vi "索引数据并插入.vi"(8 "error in (no error)":errorcluster, 9 "数据类别":enum16{"水样数据", "日质控数据"}(ring), 10 "索引记录":timestamp format="%<%H:%M:%S\n%m/%d/%Y>T", 11 "table":string) -> (0 "error out":errorcluster, 3 "最新索引记录":timestamp)   [LabVIEW 2016, in "数据查询.lvlib"]
uses:
  <vilib>/addons/database/Connection.llb/DB Tools Open Connec (String).vi
  <vilib>/addons/database/_DB Variant To Data/Database Variant To Data.xnode
  <vilib>/addons/database/NI_Database_API.lvlib
panel:
  in  "data in":cluster{"时间":timestamp, "测量模式":string, "值":sgl}
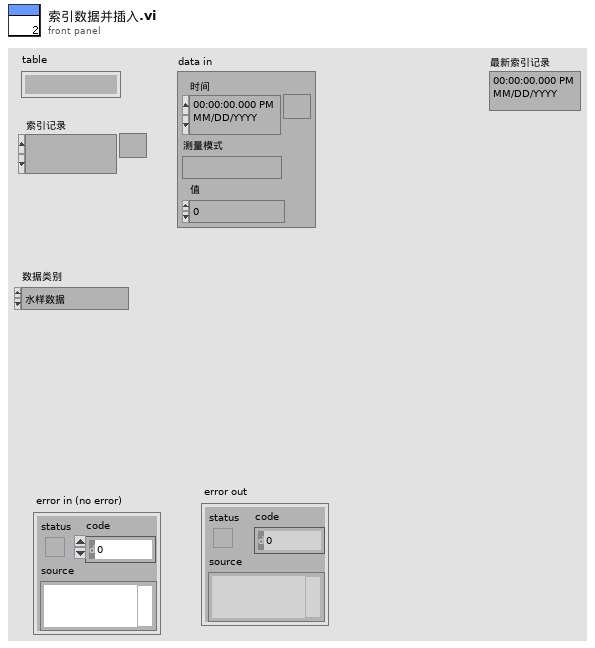
[diagram p1: front panel]
types:
  T1 = typedef "数据库类型.ctl" = enum16{"Access", "SQLite"}
  T2 = cluster{"时间":timestamp, "测量模式":string, "值":sgl}[]
  T3 = typedef "NI_Database_API.lvlib/Conn ObjectReference.ctl" = refnum<k1>
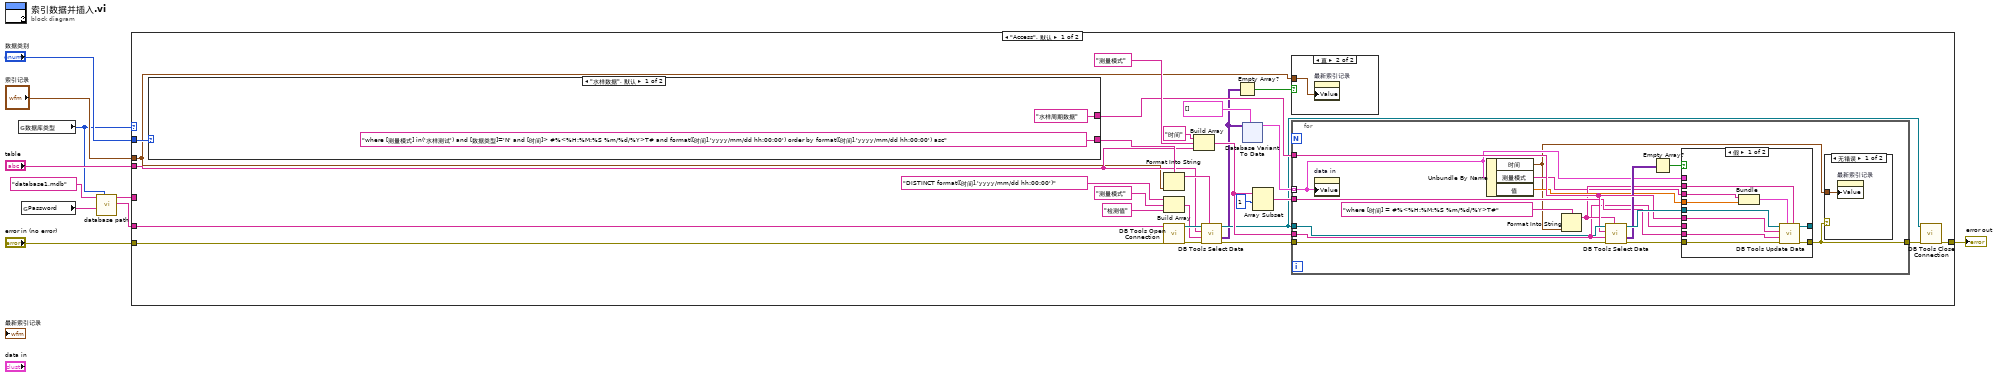
[diagram p0: block diagram]
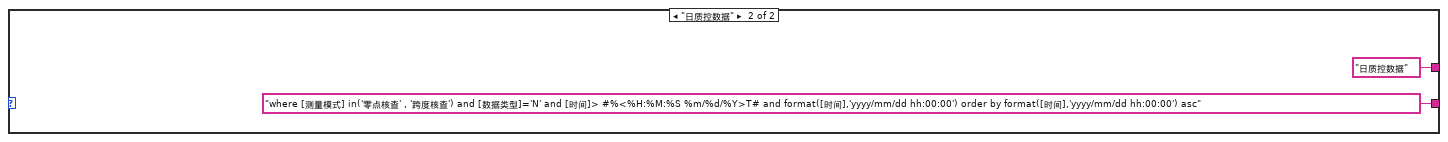
[diagram p3: hidden frame]
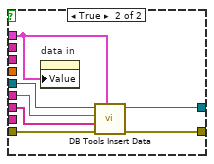
[diagram p5: hidden frame]
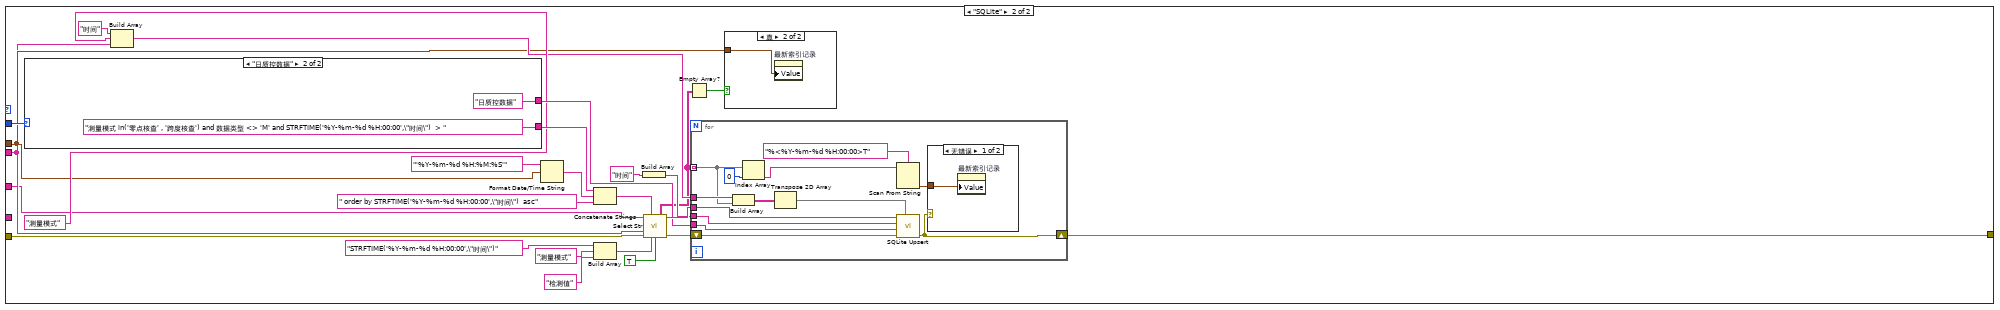
[diagram p6: hidden frame]
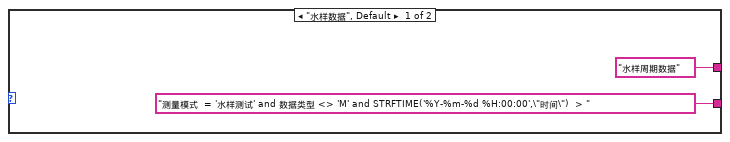
[diagram p9: hidden frame]
diagram:
  n1 = global read "全局变量.vi" "数据库类型"() -> (w4:T1)
  n2 = global read "全局变量.vi" "Password"() -> (w1:string)
  n3 = call "database path.vi"("数据库类型"=w4, "Password"=w1, "database"="database1.mdb") -> ("Connection information"=w2:string, "Path out"=w3:string)  [unwired: 7 in]
  n4 = case shown="\"Access\", 默认" w4 {
    tunnel: "索引记录" -> [w13 w195]
    tunnel: "error in (no error)" -> [w28 w217]
    tunnel: [w27 w201] -> w6
    tunnel: "数据类别" -> [w21 w218]
    tunnel: "table" -> [w20 w194]
    tunnel: w3 -> [_ w193]
    tunnel: w2 -> [w11 _]
    frame "Access", Default {
      n5 = case shown="\"水样数据\", 默认" w21 {
        tunnel: ["where [测量模式] in('水样测试') and [数据类型]='N' and [时间]> #%<%H:%M:%S %m/%d/%Y>T# and format([时间],'yyyy/mm/dd hh:00:00') order by format([时间],'yyyy/mm/dd hh:00:00') asc" ("condition") "where [测量模式] in('零点核查' , '跨度核查') and [数据类型]='N' and [时间]> #%<%H:%M:%S %m/%d/%Y>T# and format([时间],'yyyy/mm/dd hh:00:00') order by format([时间],'yyyy/mm/dd hh:00:00') asc" ("condition")] -> w23
        tunnel: ["水样周期数据" "日质控数据"] -> w22
        frame "水样数据", Default {
        }
        frame "日质控数据" {
        }
      }
      n6 = Format Into String(format string=w23, w13) -> (resulting string=w33:string)  [unwired: 2 in, 1 out]
      n7 = Build Array("DISTINCT format([时间],'yyyy/mm/dd hh:00:00')", "测量模式" ("元素"), "检测值" ("元素")) -> (w32:string[])
      n8 = call-poly <vilib>:"DB Tools Open Connection.vi"("error in (no error)"=w28, "connection information"=w11) -> ("error out"=w34:errorcluster, "connection reference"=w35:T3)  [unwired: 6 in]
      n9 = Build Array("时间", "测量模式" ("元素"), w20) -> (w31:string[])
      n10 = call <vilib>:"DB Tools Select Data.vi"("condition"=w33, "error in (no error)"=w34, "columns"=w32, "table"=w20, "connection reference"=w35) -> ("error out"=w16:errorcluster, "data"=w14:variant[][], "connection reference out"=w17:T3)  [unwired: 1 in]
      n11 = Empty Array?(array=w14) -> (empty?=w12:bool)
      n12 = xnode "Database Variant To Data"("database variant"=w14, "type"=T2 []) -> ("data"=w18:T2)  [unwired: 1 in, 1 out]
      n13 = Array Subset(array=w31, index=1 ("索引")) -> (w29:string[])  [unwired: 1 in]
      n14 = case shown="真" w12 {
        tunnel: w13 -> [_ w38]
        frame False {
        }
        frame True {
          n15 = property on="最新索引记录" class="AbsTime (严格)"("Value"=w38) -> ()  [unwired: 2 in, 2 out]
        }
      }
      n16 = for {
        tunnel: w18 -> [w45] mode=indexing
        tunnel: w17 -> [w56]
        tunnel: w16 -> [w55]
        tunnel: [w44] -> w15
        tunnel: w22 -> [w52]
        tunnel: w31 -> [w47]
        tunnel: w29 -> [w49]
        n17 = property on="data in" class="Clust (严格)"("Value"=w45) -> ()  [unwired: 2 in, 2 out]
        n18 = Unbundle By Name(w45) -> ("时间"=w43:timestamp, "测量模式"=w46:string, "值"=w50:sgl)
        n19 = Format Into String(format string="where [时间] = #%<%H:%M:%S %m/%d/%Y>T#" ("condition"), w43) -> (resulting string=w48:string)  [unwired: 2 in, 1 out]
        n20 = call <vilib>:"DB Tools Select Data.vi"("condition"=w48, "error in (no error)"=w55, "columns"=w47, "table"=w52, "connection reference"=w56) -> ("error out"=w53:errorcluster, "data"=w51:variant[][], "connection reference out"=w54:T3)  [unwired: 1 in]
        n21 = Empty Array?(array=w51) -> (empty?=w57:bool)
        n22 = case shown="假" w57 {
          tunnel: w52 -> [w65 w76]
          tunnel: w54 -> [w69 w75]
          tunnel: w53 -> [w68 w74]
          tunnel: [w66 w72] -> w44
          tunnel: [w67 w73] -> _
          tunnel: w50 -> [w64 _]
          tunnel: w49 -> [w62 _]
          tunnel: w48 -> [w61 _]
          tunnel: w47 -> [_ w71]
          tunnel: w46 -> [w60 _]
          tunnel: w45 -> [_ w70]
          frame False {
            n23 = Bundle("测量模式"=w60, "值"=w64) -> (w63:cluster{"测量模式":string, "值":sgl})  [unwired: 1 in]
            n24 = call <vilib>:"DB Tools Update Data.vi"("condition"=w61, "data"=w63, "error in (no error)"=w68, "columns"=w62, "table"=w65, "connection reference"=w69) -> ("error out"=w66:errorcluster, "connection reference out"=w67:T3)  [unwired: 4 in]
          }
          frame True {
            n25 = property on="data in" class="Clust (严格)"("Value"=w70) -> ()  [unwired: 2 in, 2 out]
            n26 = call <vilib>:"DB Tools Insert Data.vi"("data"=w70, "error in (no error)"=w74, "columns"=w71, "table"=w76, "connection reference"=w75) -> ("error out"=w72:errorcluster, "connection reference out"=w73:T3)  [unwired: 5 in]
          }
        }
        n27 = case shown="无错误" w44 {
          tunnel: w43 -> [w59 _]
          frame No Error {
            n28 = property on="最新索引记录" class="AbsTime (严格)"("Value"=w59) -> ()  [unwired: 2 in, 2 out]
          }
          frame Error {
          }
        }
      }
      n29 = call <vilib>:"DB Tools Close Connection.vi"("error in (no error)"=w15, "connection reference"=w17) -> ("error out"=w27:errorcluster)  [unwired: 5 in]
    }
    frame "SQLite" {
      n30 = case shown="\"日质控数据\"" w218 {
        tunnel: ["测量模式  = '水样测试' and 数据类型 <> 'M' and STRFTIME('%Y-%m-%d %H:00:00',\"时间\")  > " ("condition") "测量模式 in('零点核查' , '跨度核查') and 数据类型 <> 'M' and STRFTIME('%Y-%m-%d %H:00:00',\"时间\")  > " ("condition")] -> w210
        tunnel: ["水样周期数据" "日质控数据"] -> w204
        frame "水样数据", Default {
        }
        frame "日质控数据" {
        }
      }
      n31 = Build Array("时间", "测量模式" ("元素"), w194) -> (w200:string[])
      n32 = Format Date/Time String(time format string (%c)="'%Y-%m-%d %H:%M:%S'" ("时间格式字符串(%c)"), seconds (now)=w195) -> (date/time string=w209:string)  [unwired: 1 in]
      n33 = Concatenate Strings(w210, w209, " order by STRFTIME('%Y-%m-%d %H:00:00',\"时间\")  asc" ("字符串")) -> (w207:string)
      n34 = Build Array("STRFTIME('%Y-%m-%d %H:00:00',\"时间\")", "测量模式" ("元素"), "检测值" ("元素")) -> (w213:string[])
      n35 = Build Array("时间") -> (w198:string[])
      n36 = call "Select Str.vi"("DB Path"=w193, "Where Clause"=w207, "Tables Name"=w194, "error in (no error)"=w217, "Columns"=w213, "Distinct"=TRUE) -> ("Results"=w197:string[][], "DB Path Out"=w205:string, "error out"=w206:errorcluster)  [unwired: 6 in, 1 out]
      n37 = Empty Array?(array=w197) -> (empty?=w196:bool)
      n38 = for {
        tunnel: w205 -> [w222]
        tunnel: w204 -> [w220]
        tunnel: w197 -> [w229] mode=indexing
        tunnel: w200 -> [w231]
        shift-right: [w224] -> w201
        shift-left: w206 -> [w232]
        tunnel: w198 -> [w221]
        n39 = Build Array(w231, w229) -> (w230:string[][])
        n40 = Index Array(array=w229, index=0 ("索引")) -> (element=w226:string)
        n41 = Transpose 2D Array(2D array=w230) -> (transposed array=w223:string[][])
        n42 = Scan From String(format string="%<%Y-%m-%d %H:00:00>T" ("格式字符串"), input string=w226) -> (output 1=w225:timestamp)  [unwired: 3 in, 3 out]
        n43 = call "SQLite Upsert.vi"("Column/Value Pairs"=w223, "错误输入（无错误）"=w232, "Table Name"=w220, "Constraint Columns"=w221, "DB Path"=w222) -> ("错误输出"=w224:errorcluster)  [unwired: 2 in, 2 out]
        n44 = case shown="无错误" w224 {
          tunnel: w225 -> [w233 _]
          frame No Error {
            n45 = property on="最新索引记录" class="AbsTime (严格)"("Value"=w233) -> ()  [unwired: 2 in, 2 out]
          }
          frame Error {
          }
        }
      }
      n46 = case shown="真" w196 {
        tunnel: w195 -> [_ w219]
        frame False {
        }
        frame True {
          n47 = property on="最新索引记录" class="AbsTime (严格)"("Value"=w219) -> ()  [unwired: 2 in, 2 out]
        }
      }
    }
  }
  "error out" <- w6
